vi "Main - Call and Monitor TCP Traffic.vi"() -> ()   [LabVIEW 2014]
uses:
  user.lib/_NEVSTOP/Communicable State Machine(CSM)/_Support/Priority Queue/Priority Queue.lvclass/Priority Queue.ctl
  user.lib/_NEVSTOP/Communicable State Machine(CSM)/Utility/Build Error Cluster.vi
  user.lib/_NEVSTOP/Communicable State Machine(CSM)/Utility/uuid.vi
  user.lib/_NEVSTOP/Communicable State Machine(CSM)/_Support/Process/CSMP-Async Call.vi
  user.lib/_NEVSTOP/Communicable State Machine(CSM)/Utility/Trim Both Whitespace.vi
  user.lib/_NEVSTOP/Communicable State Machine(CSM)/_Support/Process/CSMP-Sync Call.vi
  user.lib/_NEVSTOP/Communicable State Machine(CSM)/_Support/CSMQ/_CSMObj-Message Check.vi
  user.lib/_NEVSTOP/Communicable State Machine(CSM)/_Support/CSMQ/_CSMObj-Enqueue Cross-Module Message.vi
  user.lib/_NEVSTOP/Communicable State Machine(CSM)/_Support/CSMQ/_CSMOFGV Get.vi
  user.lib/_NEVSTOP/Communicable State Machine(CSM)/_Support/Priority Queue/Enqueue Element.vi
  user.lib/_NEVSTOP/Communicable State Machine(CSM)/_Support/CSMQ/_CSMOFGV.vi
  user.lib/_NEVSTOP/Communicable State Machine(CSM)/Communicable State Machine.lvlib
panel:
  in  "String":string
  out "String Cache":string
  # "Overview:\n\nDemonstrates how to invoke the CSM submodule a side loop. Externally, this process is indistinguishable from other submodules based on CSM. What requires attention are the API and status changes.\n\nInstructions::\n\n1. Run this VI.\n2. Run the slightly modified Simple TCP - Client.vi, which is based on the LabVIEW example.\n3. Modify the String control on both this front panel and the client, and observe the log information.\n4. You can restart Simple TCP - Client.vi to view the logs."
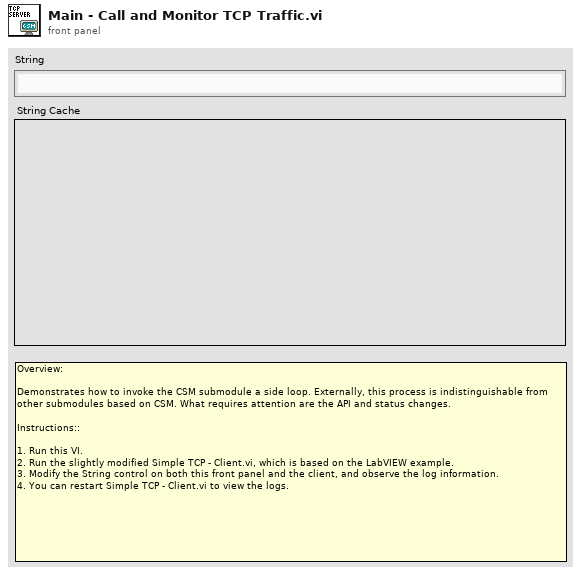
[diagram p1: front panel]
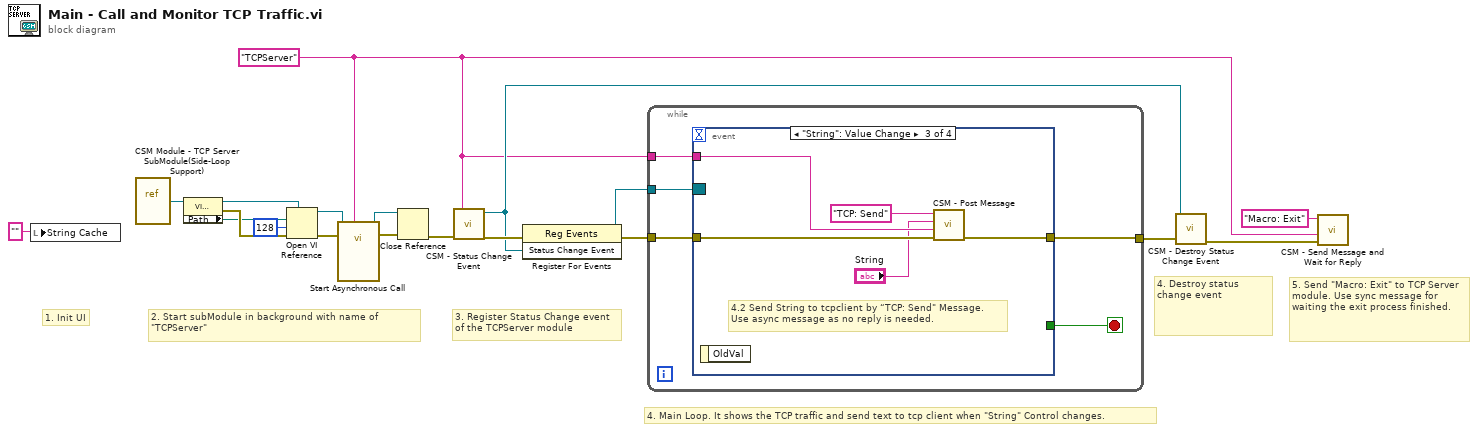
[diagram p0: block diagram]
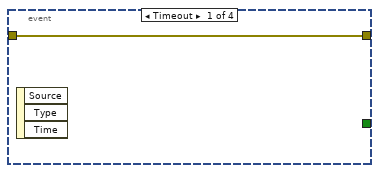
[diagram p2: hidden frame]
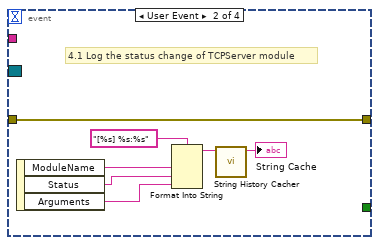
[diagram p3: hidden frame]
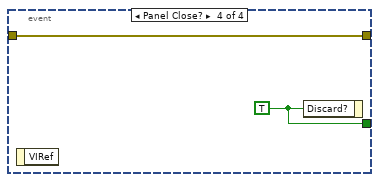
[diagram p4: hidden frame]
diagram:
  w3 = "TCPServer" ("Name(\"\" to use uuid)")
  # "5. Send \"Macro: Exit\" to TCP Server module. Use sync message for waiting the exit process finished."
  # "4. Destroy status change event"
  # "4. Main Loop. It shows the TCP traffic and send text to tcp client when \"String\" Control changes."
  # "3. Register Status Change event\nof the TCPServer module"
  # "2. Start subModule in background with name of \"TCPServer\""
  # "1. Init UI"
  n1 = local write "String Cache"("" ("String Cache")) -> ()
  n2 = vi-ref "CSM Module - TCP Server SubModule(Side-Loop Support).vi"() -> (w12:refnum<vi>)
  n3 = property class="VI (strict)"(reference=w12) -> (reference out=w16:refnum<vi>, error out=w14:errorcluster, "Path"=w13:path)  [unwired: 1 in]
  n4 = Open VI Reference(type specifier VI Refnum (for type only)=w16, vi path=w13, options=128, error in (no error)=w14) -> (vi reference=w15:refnum<vi>, error out=w11:errorcluster)  [unwired: 2 in]
  n5 = call-by-ref "Start Asynchronous Call"(reference=w15, error in=w11, "Name(\"\" to use uuid)"=w3) -> (reference out=w18:refnum<vi>, error out=w17:errorcluster)  [unwired: 11 in]
  n6 = Close Reference(reference=w18, error in (no error)=w17) -> (error out=w10:errorcluster)
  n7 = call "CSM - Status Change Event.vi"("Error in"=w10, "Name(\"\" to use uuid) in"=w3) -> ("Error out"=w9:errorcluster, "Status Change Event"=w5:refnum<user-event>)  [unwired: 8 in]
  n8 = register-events(error in=w9, w5) -> (reference out=w7:refnum<event-registration>, error out=w8:errorcluster)  [unwired: 1 in]
  n9 = while {
    tunnel: w8 -> [w21]
    tunnel: w7 -> [w23]
    tunnel: [w22] -> w6
    tunnel: w3 -> [w20]
    stop <- w24 stop-if-true
    n10 = event shown="[2] \"String\": Value Change" {
      selector: w23 -> [_ _ _ _]
      dyn-events: _ -> [_ _ _ _]
      timeout: _ -> [_ _ _ _]
      tunnel: [_ _ _ w39] -> w24
      tunnel: [w25 w32 w36 w38] -> w22
      tunnel: w21 -> [w25 w32 w37 w38]
      tunnel: w20 -> [_ _ w35 _]
      event Timeout {
        n11 = event-data() -> ()  [unwired: 1 in, 3 out]
      }
      event User Event {
        # "4.1 Log the status change of TCPServer module"
        n12 = event-data() -> ("ModuleName"=w31:string, "Status"=w30:string, "Arguments"=w29:string)  [unwired: 1 in]
        n13 = Format Into String(format string="[%s] %s:%s", w31, w30, w29) -> (resulting string=w27:string)  [unwired: 2 in, 1 out]
        n14 = call "String History Cacher.vi"("String"=w27) -> ("String Cache"=→"String Cache":string)  [unwired: 10 in]
      }
      event "String": Value Change {
        # "4.2 Send String to tcpclient by “TCP: Send\" Message.\nUse async message as no reply is needed."
        n15 = event-data() -> ()  [unwired: 1 in, 1 out]
        n16 = call "CSM - Post Message.vi"("Error In (no error)"=w37, "Target Module"=w35, "Arguments (\"\")"="String", "State"="TCP: Send") -> ("error out"=w36:errorcluster)  [unwired: 7 in]
      }
      event Panel Close? {
        w39 = TRUE ("Discard?")
        n17 = event-data() -> ()  [unwired: 1 in, 1 out]
        n18 = event-data("Discard?"=w39) -> ()  [unwired: 1 in, 1 out]
      }
    }
  }
  n19 = call "CSM - Destroy Status Change Event.vi"("Error in"=w6, "Status Change Event"=w5) -> ("Error out"=w4:errorcluster)  [unwired: 9 in]
  n20 = call "CSM - Send Message and Wait for Reply.vi"("Error In (no error)"=w4, "Target Module"=w3, "State"="Macro: Exit") -> ()  [unwired: 6 in, 3 out]
